vi "SpectrumAnn SCPI commands.vi"(11 "Path":path) -> (0 "error out":errorcluster, 2 "result string":string="3-19-2018", 3 "VISA Refnum out":refnum<visa-resource-name>)   [LabVIEW 2017]
uses:
  <vilib>/regexp/Match Regular Expression.xnode
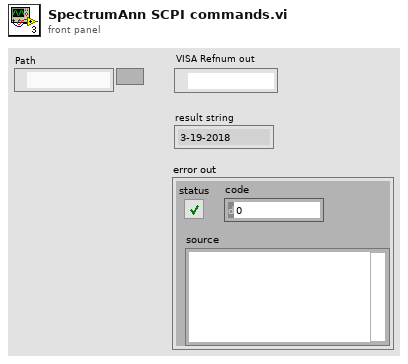
[diagram p1: front panel]
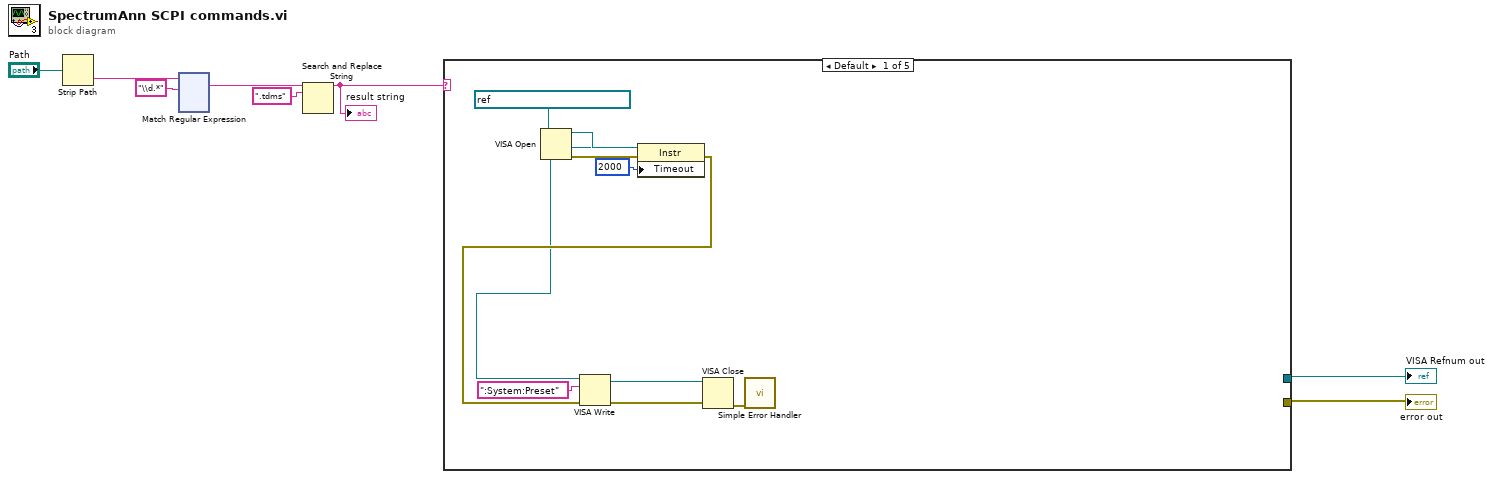
[diagram p0: block diagram]
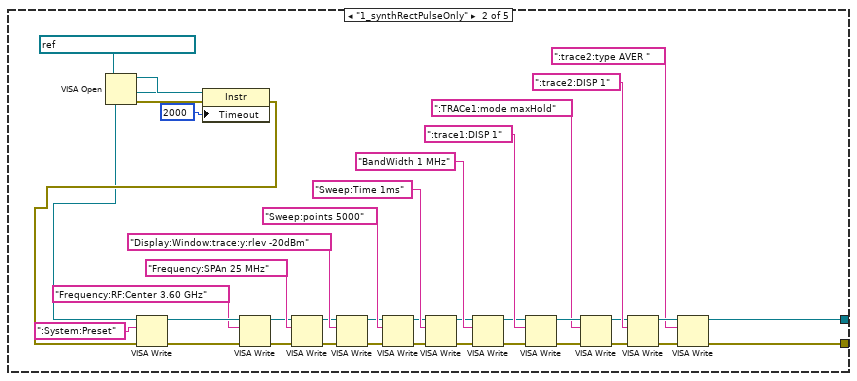
[diagram p2: hidden frame]
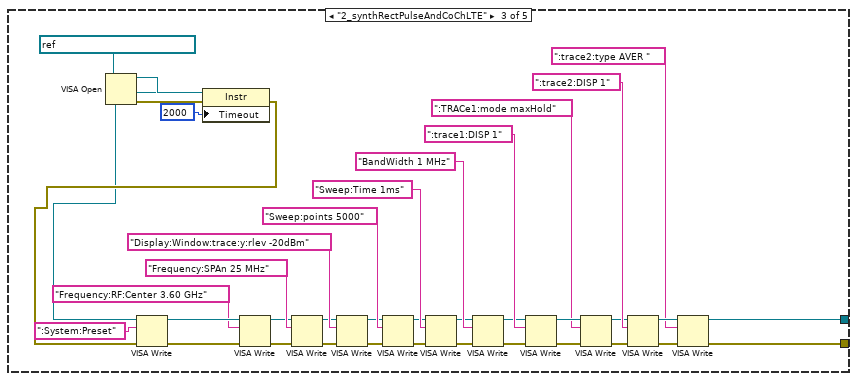
[diagram p3: hidden frame]
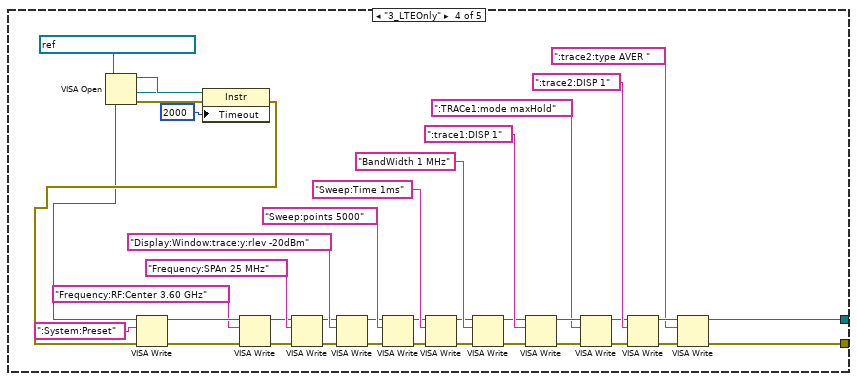
[diagram p4: hidden frame]
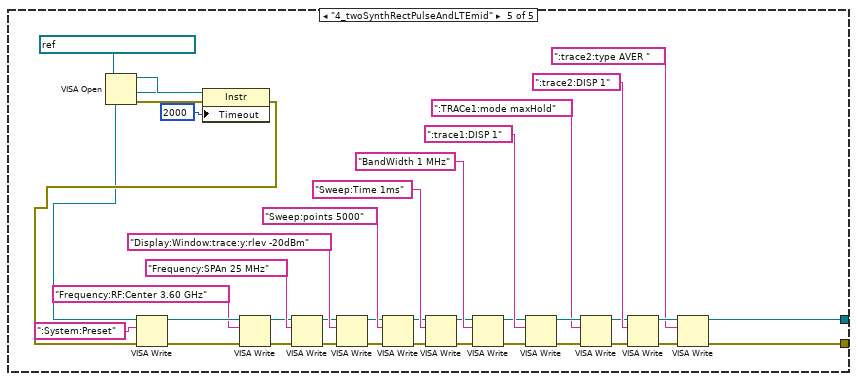
[diagram p5: hidden frame]
diagram:
  n1 = Strip Path(path="Path") -> (name=w5:string)  [unwired: 1 out]
  n2 = xnode "Match Regular Expression"("input string"=w5, "regular expression"="\\d.*") -> ("whole match"=w1:string)  [unwired: 4 in, 4 out]
  n3 = Search and Replace String(input string=w1, search string=".tdms") -> (result string=w6:string)  [unwired: 6 in, 3 out]
  "result string" <- w6
  n4 = case shown="Default" w6 {
    tunnel: [_ w25 w64 w103 w142] -> w7
    tunnel: [_ w26 w65 w104 w143] -> w8
    frame Default {
      n5 = VISA Open(VISA resource name=refnum<visa-resource-name> "SpecAnn-9010A-20100") -> (VISA resource name=w16:refnum<visa-resource-name>, error out=w15:errorcluster)  [unwired: 4 in]
      n6 = property class="Instr"(reference=w16, error in=w15, "Timeout"=u32 2000 ("General Settings:Timeout Value")) -> (reference out=w12:refnum<visa-resource-name>, error out=w13:errorcluster)
      n7 = VISA Write(VISA resource name=w12, write buffer=":System:Preset", error in (no error)=w13) -> (VISA resource name out=w10:refnum<visa-resource-name>, error out=w9:errorcluster)  [unwired: 1 out]
      n8 = VISA Close(VISA resource name=w10, error in (no error)=w9) -> (error out=w11:errorcluster)
      n9 = call <vilib>:"Simple Error Handler.vi"("error in (no error)"=w11) -> ()  [unwired: 4 in, 5 out]
    }
    frame "1_synthRectPulseOnly" {
      n10 = VISA Open(VISA resource name=refnum<visa-resource-name> "SpecAnn-9010A-20100") -> (VISA resource name=w23:refnum<visa-resource-name>, error out=w22:errorcluster)  [unwired: 4 in]
      n11 = property class="Instr"(reference=w23, error in=w22, "Timeout"=u32 2000 ("General Settings:Timeout Value")) -> (reference out=w19:refnum<visa-resource-name>, error out=w20:errorcluster)
      n12 = VISA Write(VISA resource name=w19, write buffer=":System:Preset", error in (no error)=w20) -> (VISA resource name out=w47:refnum<visa-resource-name>, error out=w46:errorcluster)  [unwired: 1 out]
      n13 = VISA Write(VISA resource name=w47, write buffer="Frequency:RF:Center 3.60 GHz", error in (no error)=w46) -> (VISA resource name out=w39:refnum<visa-resource-name>, error out=w30:errorcluster)  [unwired: 1 out]
      n14 = VISA Write(VISA resource name=w39, write buffer="Frequency:SPAn 25 MHz", error in (no error)=w30) -> (VISA resource name out=w38:refnum<visa-resource-name>, error out=w31:errorcluster)  [unwired: 1 out]
      n15 = VISA Write(VISA resource name=w38, write buffer="Display:Window:trace:y:rlev -20dBm", error in (no error)=w31) -> (VISA resource name out=w37:refnum<visa-resource-name>, error out=w32:errorcluster)  [unwired: 1 out]
      n16 = VISA Write(VISA resource name=w37, write buffer="Sweep:points 5000", error in (no error)=w32) -> (VISA resource name out=w36:refnum<visa-resource-name>, error out=w33:errorcluster)  [unwired: 1 out]
      n17 = VISA Write(VISA resource name=w36, write buffer="Sweep:Time 1ms", error in (no error)=w33) -> (VISA resource name out=w35:refnum<visa-resource-name>, error out=w34:errorcluster)  [unwired: 1 out]
      n18 = VISA Write(VISA resource name=w35, write buffer="BandWidth 1 MHz", error in (no error)=w34) -> (VISA resource name out=w28:refnum<visa-resource-name>, error out=w29:errorcluster)  [unwired: 1 out]
      n19 = VISA Write(VISA resource name=w28, write buffer=":trace1:DISP 1", error in (no error)=w29) -> (VISA resource name out=w53:refnum<visa-resource-name>, error out=w52:errorcluster)  [unwired: 1 out]
      n20 = VISA Write(VISA resource name=w53, write buffer=":TRACe1:mode maxHold", error in (no error)=w52) -> (VISA resource name out=w50:refnum<visa-resource-name>, error out=w49:errorcluster)  [unwired: 1 out]
      n21 = VISA Write(VISA resource name=w50, write buffer=":trace2:DISP 1", error in (no error)=w49) -> (VISA resource name out=w56:refnum<visa-resource-name>, error out=w57:errorcluster)  [unwired: 1 out]
      n22 = VISA Write(VISA resource name=w56, write buffer=":trace2:type AVER ", error in (no error)=w57) -> (VISA resource name out=w25:refnum<visa-resource-name>, error out=w26:errorcluster)  [unwired: 1 out]
    }
    frame "2_synthRectPulseAndCoChLTE" {
      n23 = VISA Open(VISA resource name=refnum<visa-resource-name> "SpecAnn-9010A-20100") -> (VISA resource name=w62:refnum<visa-resource-name>, error out=w61:errorcluster)  [unwired: 4 in]
      n24 = property class="Instr"(reference=w62, error in=w61, "Timeout"=u32 2000 ("General Settings:Timeout Value")) -> (reference out=w58:refnum<visa-resource-name>, error out=w59:errorcluster)
      n25 = VISA Write(VISA resource name=w58, write buffer=":System:Preset", error in (no error)=w59) -> (VISA resource name out=w86:refnum<visa-resource-name>, error out=w85:errorcluster)  [unwired: 1 out]
      n26 = VISA Write(VISA resource name=w86, write buffer="Frequency:RF:Center 3.60 GHz", error in (no error)=w85) -> (VISA resource name out=w78:refnum<visa-resource-name>, error out=w69:errorcluster)  [unwired: 1 out]
      n27 = VISA Write(VISA resource name=w78, write buffer="Frequency:SPAn 25 MHz", error in (no error)=w69) -> (VISA resource name out=w77:refnum<visa-resource-name>, error out=w70:errorcluster)  [unwired: 1 out]
      n28 = VISA Write(VISA resource name=w77, write buffer="Display:Window:trace:y:rlev -20dBm", error in (no error)=w70) -> (VISA resource name out=w76:refnum<visa-resource-name>, error out=w71:errorcluster)  [unwired: 1 out]
      n29 = VISA Write(VISA resource name=w76, write buffer="Sweep:points 5000", error in (no error)=w71) -> (VISA resource name out=w75:refnum<visa-resource-name>, error out=w72:errorcluster)  [unwired: 1 out]
      n30 = VISA Write(VISA resource name=w75, write buffer="Sweep:Time 1ms", error in (no error)=w72) -> (VISA resource name out=w74:refnum<visa-resource-name>, error out=w73:errorcluster)  [unwired: 1 out]
      n31 = VISA Write(VISA resource name=w74, write buffer="BandWidth 1 MHz", error in (no error)=w73) -> (VISA resource name out=w67:refnum<visa-resource-name>, error out=w68:errorcluster)  [unwired: 1 out]
      n32 = VISA Write(VISA resource name=w67, write buffer=":trace1:DISP 1", error in (no error)=w68) -> (VISA resource name out=w92:refnum<visa-resource-name>, error out=w91:errorcluster)  [unwired: 1 out]
      n33 = VISA Write(VISA resource name=w92, write buffer=":TRACe1:mode maxHold", error in (no error)=w91) -> (VISA resource name out=w89:refnum<visa-resource-name>, error out=w88:errorcluster)  [unwired: 1 out]
      n34 = VISA Write(VISA resource name=w89, write buffer=":trace2:DISP 1", error in (no error)=w88) -> (VISA resource name out=w95:refnum<visa-resource-name>, error out=w96:errorcluster)  [unwired: 1 out]
      n35 = VISA Write(VISA resource name=w95, write buffer=":trace2:type AVER ", error in (no error)=w96) -> (VISA resource name out=w64:refnum<visa-resource-name>, error out=w65:errorcluster)  [unwired: 1 out]
    }
    frame "3_LTEOnly" {
      n36 = VISA Open(VISA resource name=refnum<visa-resource-name> "SpecAnn-9010A-20100") -> (VISA resource name=w101:refnum<visa-resource-name>, error out=w100:errorcluster)  [unwired: 4 in]
      n37 = property class="Instr"(reference=w101, error in=w100, "Timeout"=u32 2000 ("General Settings:Timeout Value")) -> (reference out=w97:refnum<visa-resource-name>, error out=w98:errorcluster)
      n38 = VISA Write(VISA resource name=w97, write buffer=":System:Preset", error in (no error)=w98) -> (VISA resource name out=w125:refnum<visa-resource-name>, error out=w124:errorcluster)  [unwired: 1 out]
      n39 = VISA Write(VISA resource name=w125, write buffer="Frequency:RF:Center 3.60 GHz", error in (no error)=w124) -> (VISA resource name out=w117:refnum<visa-resource-name>, error out=w108:errorcluster)  [unwired: 1 out]
      n40 = VISA Write(VISA resource name=w117, write buffer="Frequency:SPAn 25 MHz", error in (no error)=w108) -> (VISA resource name out=w116:refnum<visa-resource-name>, error out=w109:errorcluster)  [unwired: 1 out]
      n41 = VISA Write(VISA resource name=w116, write buffer="Display:Window:trace:y:rlev -20dBm", error in (no error)=w109) -> (VISA resource name out=w115:refnum<visa-resource-name>, error out=w110:errorcluster)  [unwired: 1 out]
      n42 = VISA Write(VISA resource name=w115, write buffer="Sweep:points 5000", error in (no error)=w110) -> (VISA resource name out=w114:refnum<visa-resource-name>, error out=w111:errorcluster)  [unwired: 1 out]
      n43 = VISA Write(VISA resource name=w114, write buffer="Sweep:Time 1ms", error in (no error)=w111) -> (VISA resource name out=w113:refnum<visa-resource-name>, error out=w112:errorcluster)  [unwired: 1 out]
      n44 = VISA Write(VISA resource name=w113, write buffer="BandWidth 1 MHz", error in (no error)=w112) -> (VISA resource name out=w106:refnum<visa-resource-name>, error out=w107:errorcluster)  [unwired: 1 out]
      n45 = VISA Write(VISA resource name=w106, write buffer=":trace1:DISP 1", error in (no error)=w107) -> (VISA resource name out=w131:refnum<visa-resource-name>, error out=w130:errorcluster)  [unwired: 1 out]
      n46 = VISA Write(VISA resource name=w131, write buffer=":TRACe1:mode maxHold", error in (no error)=w130) -> (VISA resource name out=w128:refnum<visa-resource-name>, error out=w127:errorcluster)  [unwired: 1 out]
      n47 = VISA Write(VISA resource name=w128, write buffer=":trace2:DISP 1", error in (no error)=w127) -> (VISA resource name out=w134:refnum<visa-resource-name>, error out=w135:errorcluster)  [unwired: 1 out]
      n48 = VISA Write(VISA resource name=w134, write buffer=":trace2:type AVER ", error in (no error)=w135) -> (VISA resource name out=w103:refnum<visa-resource-name>, error out=w104:errorcluster)  [unwired: 1 out]
    }
    frame "4_twoSynthRectPulseAndLTEmid" {
      n49 = VISA Open(VISA resource name=refnum<visa-resource-name> "SpecAnn-9010A-20100") -> (VISA resource name=w140:refnum<visa-resource-name>, error out=w139:errorcluster)  [unwired: 4 in]
      n50 = property class="Instr"(reference=w140, error in=w139, "Timeout"=u32 2000 ("General Settings:Timeout Value")) -> (reference out=w136:refnum<visa-resource-name>, error out=w137:errorcluster)
      n51 = VISA Write(VISA resource name=w136, write buffer=":System:Preset", error in (no error)=w137) -> (VISA resource name out=w164:refnum<visa-resource-name>, error out=w163:errorcluster)  [unwired: 1 out]
      n52 = VISA Write(VISA resource name=w164, write buffer="Frequency:RF:Center 3.60 GHz", error in (no error)=w163) -> (VISA resource name out=w156:refnum<visa-resource-name>, error out=w147:errorcluster)  [unwired: 1 out]
      n53 = VISA Write(VISA resource name=w156, write buffer="Frequency:SPAn 25 MHz", error in (no error)=w147) -> (VISA resource name out=w155:refnum<visa-resource-name>, error out=w148:errorcluster)  [unwired: 1 out]
      n54 = VISA Write(VISA resource name=w155, write buffer="Display:Window:trace:y:rlev -20dBm", error in (no error)=w148) -> (VISA resource name out=w154:refnum<visa-resource-name>, error out=w149:errorcluster)  [unwired: 1 out]
      n55 = VISA Write(VISA resource name=w154, write buffer="Sweep:points 5000", error in (no error)=w149) -> (VISA resource name out=w153:refnum<visa-resource-name>, error out=w150:errorcluster)  [unwired: 1 out]
      n56 = VISA Write(VISA resource name=w153, write buffer="Sweep:Time 1ms", error in (no error)=w150) -> (VISA resource name out=w152:refnum<visa-resource-name>, error out=w151:errorcluster)  [unwired: 1 out]
      n57 = VISA Write(VISA resource name=w152, write buffer="BandWidth 1 MHz", error in (no error)=w151) -> (VISA resource name out=w145:refnum<visa-resource-name>, error out=w146:errorcluster)  [unwired: 1 out]
      n58 = VISA Write(VISA resource name=w145, write buffer=":trace1:DISP 1", error in (no error)=w146) -> (VISA resource name out=w170:refnum<visa-resource-name>, error out=w169:errorcluster)  [unwired: 1 out]
      n59 = VISA Write(VISA resource name=w170, write buffer=":TRACe1:mode maxHold", error in (no error)=w169) -> (VISA resource name out=w167:refnum<visa-resource-name>, error out=w166:errorcluster)  [unwired: 1 out]
      n60 = VISA Write(VISA resource name=w167, write buffer=":trace2:DISP 1", error in (no error)=w166) -> (VISA resource name out=w173:refnum<visa-resource-name>, error out=w174:errorcluster)  [unwired: 1 out]
      n61 = VISA Write(VISA resource name=w173, write buffer=":trace2:type AVER ", error in (no error)=w174) -> (VISA resource name out=w142:refnum<visa-resource-name>, error out=w143:errorcluster)  [unwired: 1 out]
    }
  }
  "error out" <- w8
  "VISA Refnum out" <- w7
